vi "Read Umgebung.Zustandsgrössen.vi"(8 "error in (no error)":errorcluster, 11 "Umgebung in":refnum<class "Umgebung.lvclass">) -> (0 "error out":errorcluster, 2 "Umgebung.Zustandsgrössen":T1, 3 "Umgebung out":refnum<class "Umgebung.lvclass">)   [LabVIEW 2016, in "Umgebung.lvclass"]
uses:
  Umgebung.lvclass
  Umgebung.lvclass/Umgebung.ctl
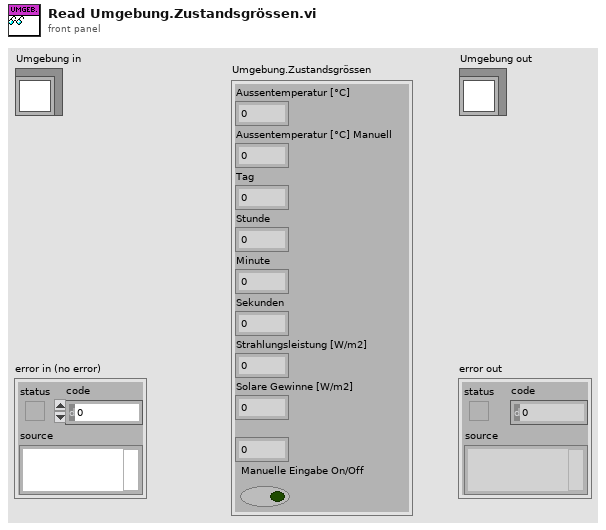
[diagram p1: front panel]
types:
  T1 = typedef "Umgebung.lvclass/Umgebung.Zustandsgrössen.ctl" = cluster{"Aussentemperatur [°C]":dbl, "Aussentemperatur [°C] Manuell":dbl, "Tag":dbl, "Stunde":dbl, "Minute":dbl, "Sekunden":dbl, "Strahlungsleistung [W/m2]":dbl, "Solare Gewinne [W/m2]":dbl, "Solare Gewinne [W/m2] Manuell":dbl, "Manuelle Eingabe On/Off":bool}
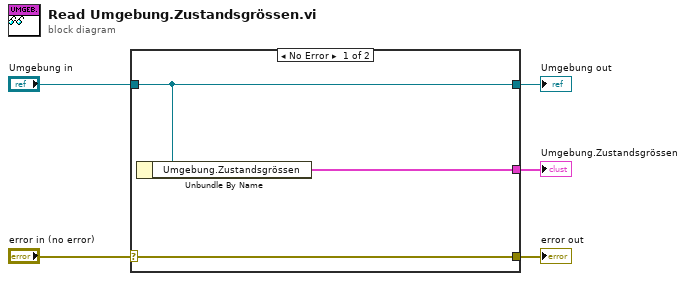
[diagram p0: block diagram]
diagram:
  n1 = case shown="No Error" "error in (no error)" {
    selector: "error in (no error)" -> [w8 w9]
    tunnel: [w8 w9] -> w4
    tunnel: [w7 w10] -> w2
    tunnel: "Umgebung in" -> [w7 w10]
    tunnel: [w6 _] -> w1
    frame No Error {
      n2 = Unbundle By Name(w7) -> ("Umgebung.Zustandsgrössen"=w6:T1)
    }
    frame Error {
    }
  }
  "error out" <- w4
  "Umgebung out" <- w2
  "Umgebung.Zustandsgrössen" <- w1
